vi "dvdg.vi"() -> ()   [LabVIEW 2017]
panel:
  in  "stop":bool
  out "Numeric Indicator":dbl
  in  "Boolean":bool
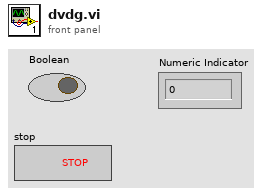
[diagram p1: front panel]
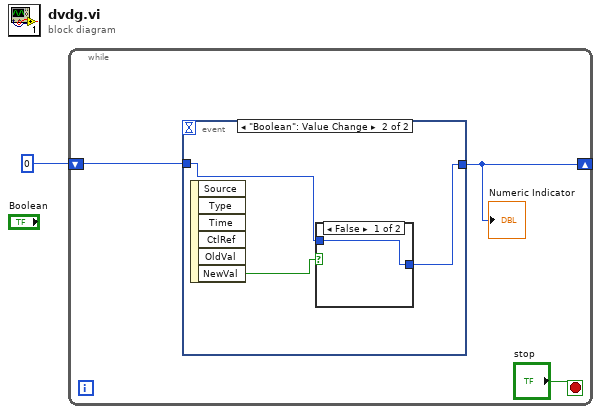
[diagram p0: block diagram]
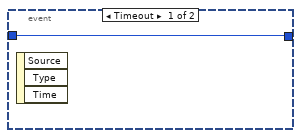
[diagram p2: hidden frame]
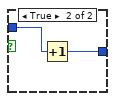
[diagram p3: hidden frame]
diagram:
  n1 = while {
    shift-right: [w3] -> _
    shift-left: 0 -> [w4]
    stop <- "stop" stop-if-true
    n2 = event shown="[1] \"Boolean\": Value Change" {
      selector: _ -> [_ _]
      dyn-events: _ -> [_ _]
      timeout: _ -> [_ _]
      tunnel: w4 -> [w5 w7]
      tunnel: [w5 w6] -> w3
      event Timeout {
        n3 = event-data() -> ()  [unwired: 1 in, 3 out]
      }
      event "Boolean": Value Change {
        n4 = event-data() -> ("NewVal"=w8:bool)  [unwired: 1 in, 5 out]
        n5 = case shown="False" w8 {
          tunnel: w7 -> [w9 w11]
          tunnel: [w9 w10] -> w6
          frame False {
          }
          frame True {
            n6 = Increment(x=w11) -> (x+1=w10:i32)
          }
        }
      }
    }
    "Numeric Indicator" <- w3
  }
